vi "Fire Alarm.vi"() -> ()   [LabVIEW 2011]
panel:
  out "error out 2":errorcluster
  in  "error in 2":errorcluster
  in  "stop":bool
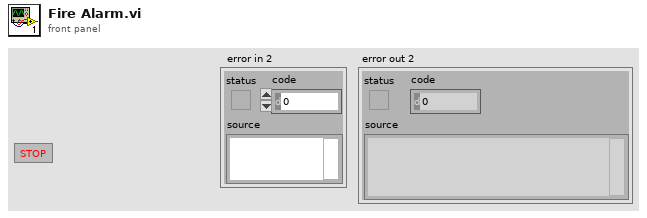
[diagram p1: front panel]
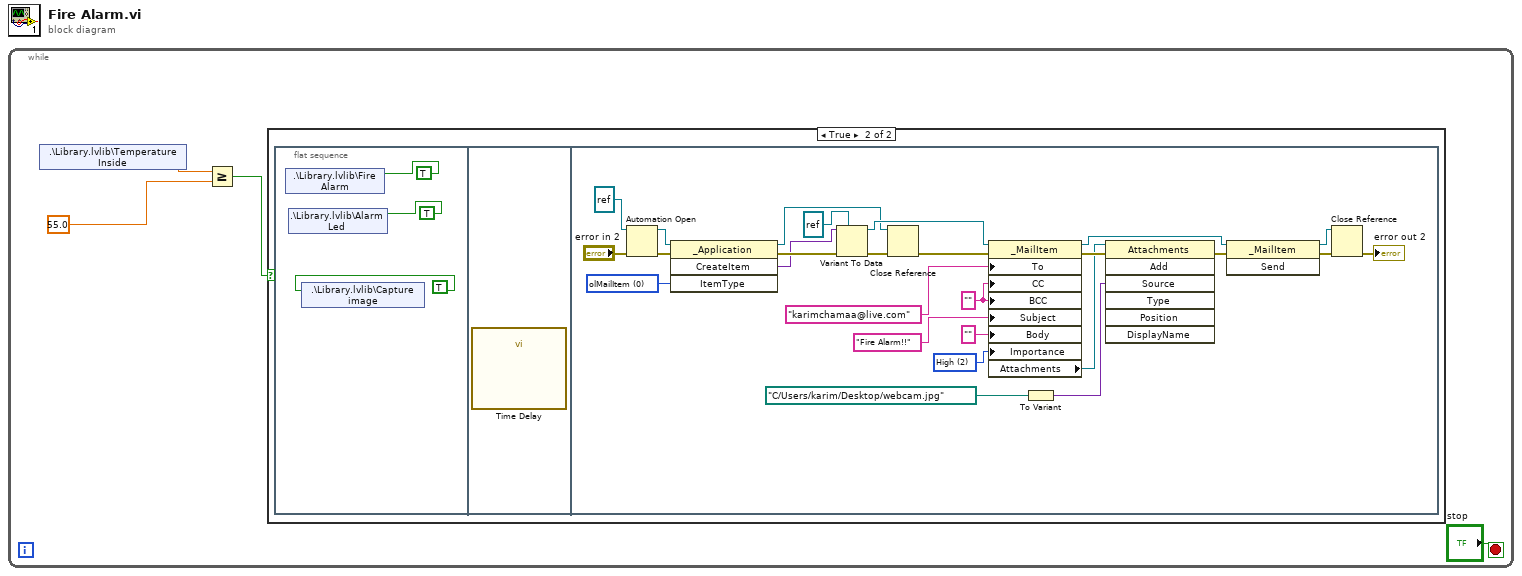
[diagram p0: block diagram]
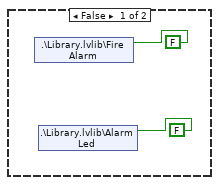
[diagram p2: hidden frame]
diagram:
  n1 = while {
    stop <- "stop" stop-if-true
    n2 = shared-variable ".\\Library.lvlib\\Temperature Inside"() -> (w3:dbl)  [unwired: 1 in, 1 out]
    n3 = Greater Or Equal?(x=w3, y=55.0) -> (x >= y?=w1:bool)
    n4 = case shown="True" w1 {
      frame False {
        n5 = shared-variable ".\\Library.lvlib\\Fire Alarm"(FALSE ("Fire Alarm")) -> ()  [unwired: 1 in, 1 out]
        n6 = shared-variable ".\\Library.lvlib\\Alarm Led"(FALSE ("Fire Alarm")) -> ()  [unwired: 1 in, 1 out]
      }
      frame True {
        n7 = flat-sequence {
          frame #0 {
            n8 = shared-variable ".\\Library.lvlib\\Fire Alarm"(TRUE ("Fire Alarm")) -> ()  [unwired: 1 in, 1 out]
            n9 = shared-variable ".\\Library.lvlib\\Alarm Led"(TRUE ("Fire Alarm")) -> ()  [unwired: 1 in, 1 out]
            n10 = shared-variable ".\\Library.lvlib\\Capture image"(TRUE ("Fire Alarm")) -> ()  [unwired: 1 in, 1 out]
          }
          frame #1 {
            n11 = call "Time Delay"() -> ()  [unwired: 11 in, 1 out]
          }
          frame #2 {
            w32 = "" ("CC")
            w31 = 2 items=["Low", "Normal", "High"] ("Importance")
            w13 = 0 items=["olMailItem", "olAppointmentItem", "olContactItem", "olTaskItem", "olJournalItem", "olNoteItem", "olPostItem"] ("ItemType")
            n12 = Automation Open(error in (no error)="error in 2", Automation Refnum=refnum<k7> refnum ("Outlook._Application")) -> (Automation Refnum=w12:refnum<k7>, error out=w19:errorcluster)  [unwired: 2 in]
            n13 = invoke class="_Application" method="CreateItem"(reference=w12, error in=w19, "ItemType"=w13) -> (reference out=w16:refnum<k7>, error out=w21:errorcluster, "CreateItem"=w14:variant)  [unwired: 1 in, 1 out]
            n14 = Variant To Data(error in=w21, type=refnum<k7> refnum ("Outlook._MailItem"), Variant=w14) -> (data=w30:refnum<k7>, error out=w22:errorcluster)
            n15 = Close Reference(reference=w16, error in (no error)=w22) -> (error out=w23:errorcluster)
            n16 = property class="_MailItem"(reference=w30, error in=w23, "To"="karimchamaa@live.com", "CC"=w32, "BCC"=w32, "Subject"="Fire Alarm!!", "Body"="" ("Message"), "Importance"=w31) -> (reference out=w29:refnum<k7>, error out=w26:errorcluster, "Attachments"=w25:refnum<k7>)
            n17 = To Variant(anything=path "C:/Users/karim/Desktop/webcam.jpg" ("Report Path")) -> (Variant=w27:variant)
            n18 = invoke class="Attachments" method="Add"(reference=w25, error in=w26, "Source"=w27) -> (error out=w28:errorcluster)  [unwired: 4 in, 6 out]
            n19 = invoke class="_MailItem" method="Send"(reference=w29, error in=w28) -> (reference out=w17:refnum<k7>, error out=w18:errorcluster)  [unwired: 1 in, 1 out]
            n20 = Close Reference(reference=w17, error in (no error)=w18) -> (error out=→"error out 2":errorcluster)
          }
        }
      }
    }
  }
